vi "Untitled 1.vi"   [LabVIEW 2025]
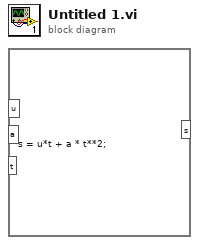
[diagram p0: block diagram]
diagram:
  n1 = formula code="s = u*t + a * t**2;"() -> ()  [unwired: 3 in, 1 out]
